vi "PH_PPMA_PowerUnit.ProcCases.vi"(0 "i ref in":refnum<vi>, 1 "selector":string, 2 "Data":T1, 3 "call cluster":T2={"Object"="", "Selector"="", "CallType"=enum."synchronous", "Async Object"="", "Async Selector"="", "Data Descriptor"="", "Data"=[], "Error #"=0, "Expire"=0}, 5 "error in (no error)":errorcluster) -> (14 "i ref out":refnum<vi>, 17 "answer cluster":T2={"Object"="", "Selector"="", "CallType"=enum."synchronous", "Async Object"="", "Async Selector"="", "Data Descriptor"="", "Data"=[], "Error #"=0, "Expire"=0}, 19 "error out":errorcluster)   [LabVIEW 2014, in "PH_PPMA_PowerUnit.lvlib"]
doc: "This method is called by a process from within the default case in the event loop. The methods of a class that are linked to events will be called from THIS method. Add your code here."
uses:
  PH_PPMA_PowerUnit.lvlib
  CSCore/CSSystem/CoreDefs/CoreDefs.call_type.ctl
  CSCore/BaseProcess/BaseProcess.descriptor string definition.ctl
  CSCore/CSSystem/CoreDefs/CoreDefs.rawDataType.ctl
  PH_PowerUnit_BaseClass/PH_PowerUnit_BaseClass.SM States.ctl
  CSCore/CSSystem/CoreLib/CoreLib.string 2 byte array.vi
  CSCore/CSSystem/CoreLib/CoreLib.byte array 2 double.vi
  CSCore/CSSystem/CoreLib/CoreLib.byte array 2 short.vi
  CSCore/CSSystem/CoreLib/CoreLib.lvlib
  CSCore/BaseProcess/BaseProcess.lvlib
  PH_Common/PH_Common.lvlib
  CSCore/CAEObj/CAEObj.lvlib
  lib.lib/DimLVEvent/LVDimInterface/LVDimInterface.lvlib
  PH_StatusHandler/PH_StatusHandler.lvlib
  PH_PSDBWriter/PH_PSDBWriter.lvlib
  CSCore/BaseSM/BaseSM.lvlib
  PH_PowerUnit_BaseClass/PH_PowerUnit_BaseClass.lvlib
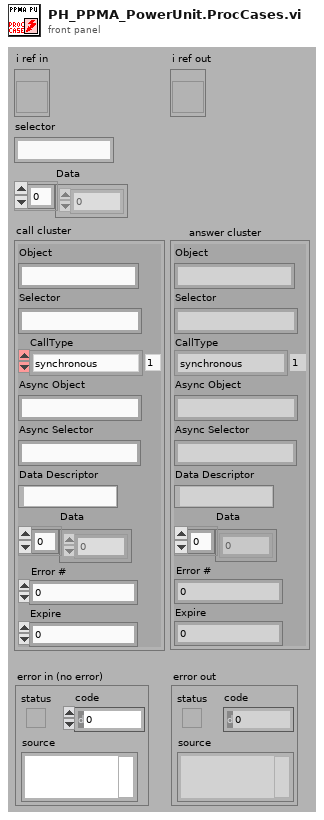
[diagram p1: front panel]
types:
  T1 = typedef "CoreDefs.rawDataType.ctl" = i8[]
  T2 = typedef "CoreDefs.call_type.ctl" = cluster{"Object":string, "Selector":string, "CallType":enum16{"simple", "synchronous", "asynchronous"}, "Async Object":string, "Async Selector":string, "Data Descriptor":T3, "Data":T1, "Error #":i32, "Expire":u32}
  T3 = typedef "BaseProcess.lvlib/BaseProcess.descriptor string definition.ctl" = string
  T4 = typedef "PH_PowerUnit_BaseClass.lvlib/PH_PowerUnit_BaseClass.SM States.ctl" = enum16{".", "Stand by", "Switch PU on", "Configure", "Set Default Voltage", "Set STANDBY", "Set READY", "Wait for Shot Cmd", "Open Dump Rods", "Open Ross Relais", "Close Ross Relais", "Switch PSU on", "Switch PSU off", "Charge", "Switch GD Channel on", "Close Dump Rods", "Rods-TO", "RR-TO", "PSU-TO", "Trigger-TO"}
  T5 = typedef "PH_PowerUnit_BaseClass.lvlib/PH_PowerUnit_BaseClass.i attribute.ctl" = cluster{"Constructor finished":bool, "PU":cluster{"In use":bool, "Service ID in use":i32, "GUI Ref":refnum<vi>}, "Enabling":cluster{"State":T6, "GUI Ref":refnum<vi>}, "Timing":cluster{"Last Shot":dbl, "Time between Shots [Sec]":dbl, "Waiting Time over?":bool, "Service ID Waiting Time":i32, "GUI Ref":refnum<vi>, "Instance":cluster{"Status":T7, "linked?":bool, "GUI Ref":refnum<vi>}}, "Sequencer":cluster{"SM State":string, "GUI Ref":refnum<vi>, "linked":bool}, "Subscribed Trendmssgs":cluster{"Tagname":string, "Status":T7, "linked?":bool, "Shot Condition":T7, "GUI Ref":refnum<vi>}[], "PP PU":T8, "Default Voltage (V)":dbl, "GUI Refs":T9, "PSDB data":cluster{"Shot Voltage [V]":dbl, "State TO SM":T4, "Write 2 early":bool}, "State TO SM":T4}
  T6 = typedef "PH_SystemInformation.lvlib/PH_SystemInformationEnabling State.ctl" = i32
  T7 = typedef "PH_StatusHandler.lvlib/PH_StatusHandler.Status.ctl" = i16
  T8 = typedef "PH_PP_Common.lvlib/PH_PP_Common.PUs.ctl" = enum16{"no Info", "PA-19mm-1", "PA-19mm-2", "PA-45mm-PILC", "PA-45mm-MAIN", "MA-PU-1", "MA-PU-2", "MA-PU-3", "MA-PU-4", "MA-PU-5", "MA-PU-6", "MA-FR", "MA-PILC", "PA-45mm-DP"}
  T9 = typedef "PH_PowerUnit_BaseClass.lvlib/PH_PowerUnit_BaseClass.GUI Refs.ctl" = cluster{"Delete Inst":refnum<vi>, "State TO SM":refnum<vi>, "State SM":refnum<vi>, "Fire":refnum<vi>}
  T10 = typedef "PH_PPMA_PowerUnit.lvlib/PH_PPMA_PowerUnit.i attribute.ctl" = cluster{"GUI Refs":cluster{"Rods":refnum<vi>, "Ignitron":refnum<vi>, "Rossrelais":refnum<vi>, "Set Voltage":refnum<vi>, "PSU":refnum<vi>, "EOC":refnum<vi>, "Trigger":refnum<vi>}, "Rods":T11, "PSU":T12, "Ross Relais":T13, "Ignitron":T14, "Trigger":cluster{"State Device":T7, "linked?":bool}, "Timing Settings":cluster{"Prdc Fast?":bool, "Default Value Periodic Interval":i32, "Mercury on since":dbl, "Warm up Time Mercury [s]":dbl}, "Set Voltage [V]":dbl}
  T11 = typedef "PH_PPMA_PowerUnit.lvlib/PH_PPMA_PowerUnit.Rods Attributes.ctl" = cluster{"Instancename":string, "Device Status":T7, "linked?":bool}
  T12 = typedef "PH_PP_Common.lvlib/PH_PP_Common.PSU Attributes.ctl" = cluster{"lower limit [V]":dbl, "upper limit [V]":dbl, "Voltage set":bool, "State Device":T7, "linked?":bool}
  T13 = typedef "PH_PP_Common.lvlib/PH_PP_Common.Ross Relais Attributes.ctl" = cluster{"State Device":T7, "linked?":bool}
  T14 = typedef "PH_PP_Common.lvlib/PH_PP_Common.Ignitron Attributes.ctl" = cluster{"State Device":T7, "linked?":bool}
  T15 = typedef "PH_PSDBWriter.lvlib/PH_PSDBWriter.PHELIX-Subsystems.ctl" = i32
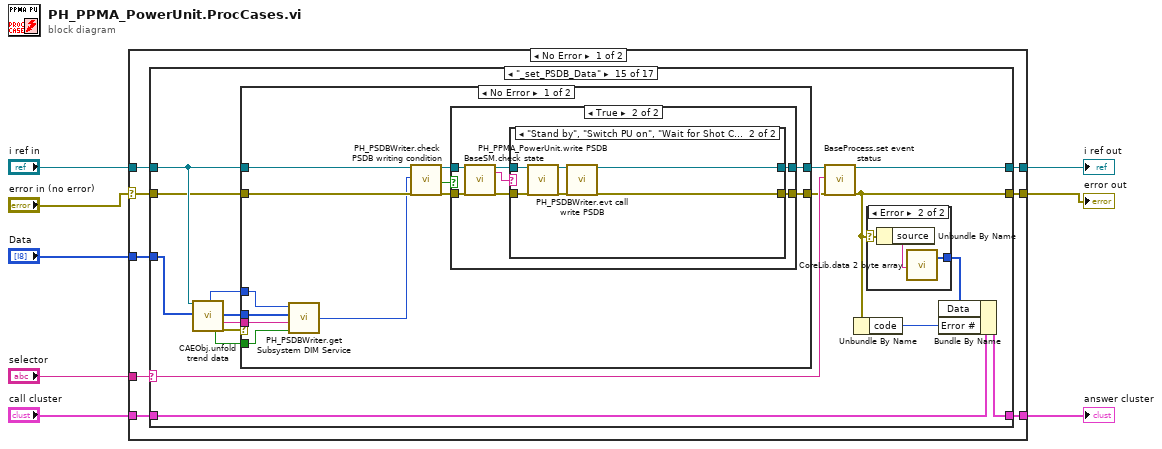
[diagram p0: block diagram]
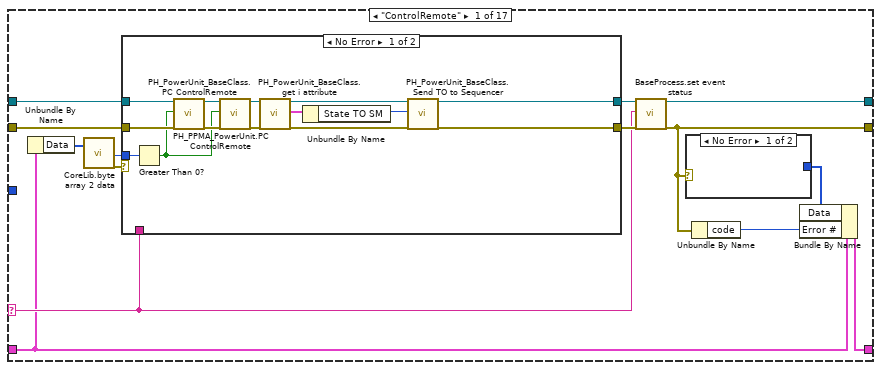
[diagram p2: hidden frame]
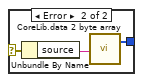
[diagram p3: hidden frame]
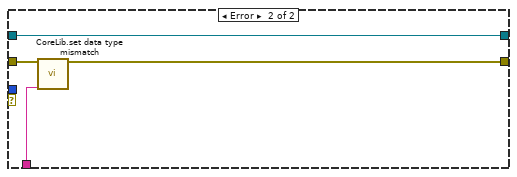
[diagram p4: hidden frame]
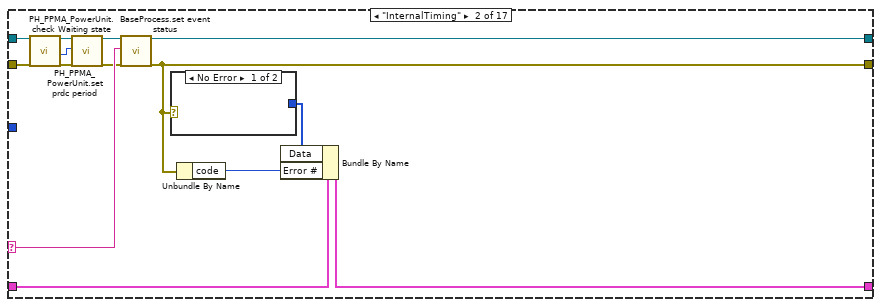
[diagram p5: hidden frame]
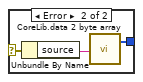
[diagram p6: hidden frame]
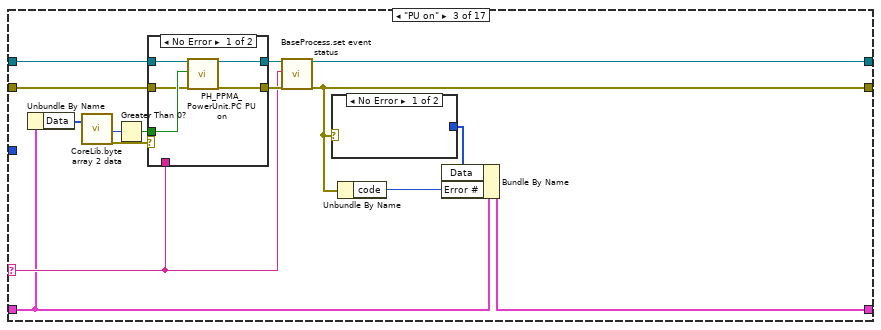
[diagram p7: hidden frame]
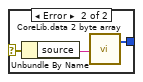
[diagram p8: hidden frame]
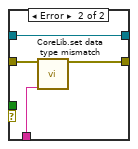
[diagram p9: hidden frame]
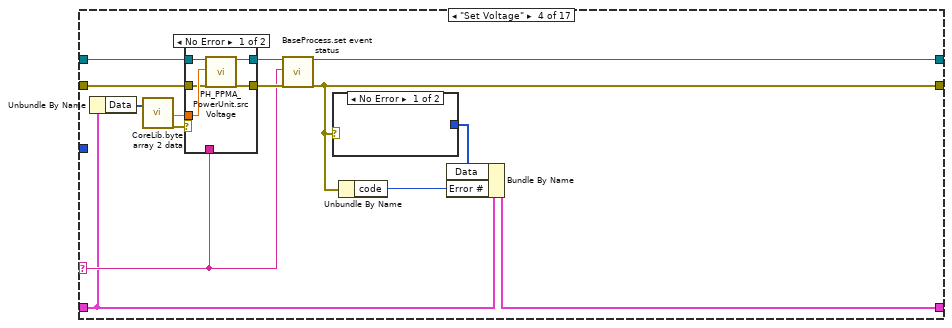
[diagram p10: hidden frame]
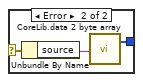
[diagram p11: hidden frame]
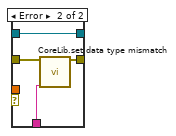
[diagram p12: hidden frame]
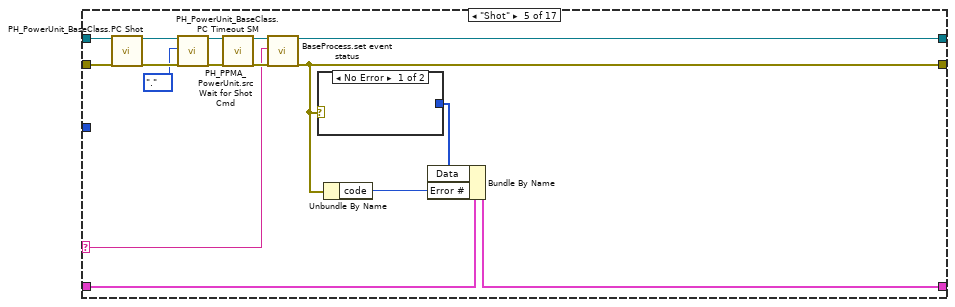
[diagram p13: hidden frame]
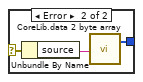
[diagram p14: hidden frame]
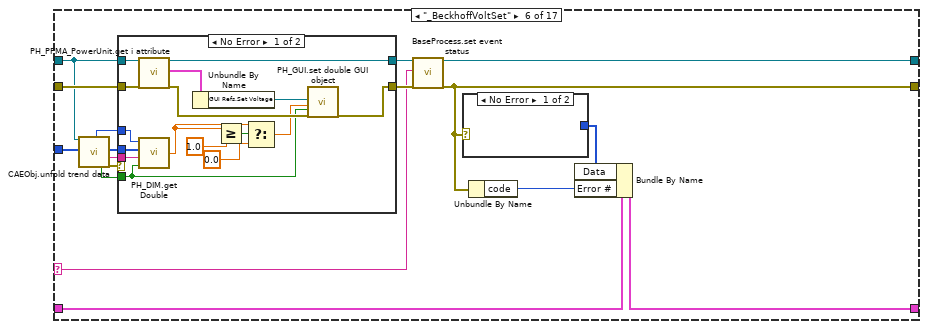
[diagram p15: hidden frame]
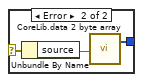
[diagram p16: hidden frame]
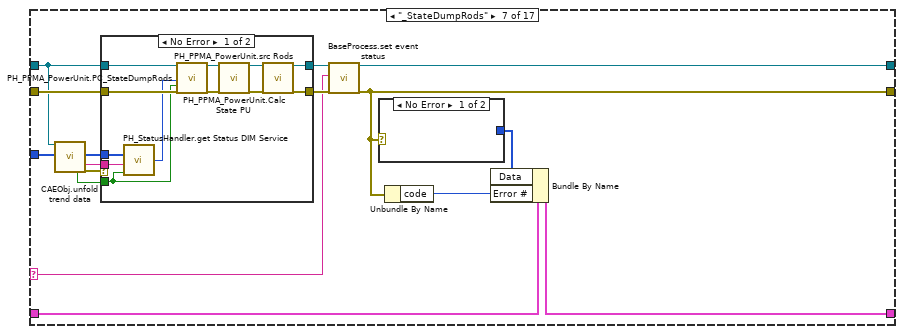
[diagram p18: hidden frame]
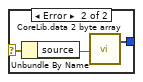
[diagram p19: hidden frame]
diagram:
  n1 = case shown="No Error" "error in (no error)" {
    selector: "error in (no error)" -> [w9 w608]
    tunnel: "selector" -> [w16 _]
    tunnel: [w15 w607] -> w7
    tunnel: "call cluster" -> [w14 w607]
    tunnel: "i ref in" -> [w13 w609]
    tunnel: [w12 w609] -> w4
    tunnel: [w11 w608] -> w3
    tunnel: "Data" -> [w10 _]
    frame No Error {
      n2 = case shown="\"_set_PSDB_Data\"" w16 {
        selector: w16 -> [w19 w61 w71 w98 w127 w143 w181 w217 w246 w299 w341 w376 w409 w444 w510 w576 w603]
        tunnel: w13 -> [w30 w56 w83 w109 w137 w155 w192 w212 w257 w310 w339 w372 w405 w437 w501 w567 w602]
        tunnel: [w21 w63 w74 w100 w123 w145 w183 w213 w248 w301 w345 w378 w411 w446 w512 w578 w599] -> w12
        tunnel: w14 -> [w18 w60 w70 w97 w126 w142 w180 w216 w245 w298 w343 w375 w408 w443 w509 w575 w604]
        tunnel: [w17 w59 w69 w96 w125 w141 w179 w215 w244 w297 w342 w374 w407 w442 w508 w574 w605] -> w15
        tunnel: w9 -> [w29 w57 w82 w108 w136 w157 w194 w227 w259 w312 w350 w383 w416 w438 w500 w566 w606]
        tunnel: [w20 w62 w72 w99 w124 w144 w182 w214 w247 w300 w344 w377 w410 w445 w511 w577 w597] -> w11
        tunnel: w10 -> [_ _ _ _ _ w156 w193 w226 w258 w311 w340 w373 w406 w434 w502 w568 w601]
        frame "ControlRemote" {
          n3 = Unbundle By Name(w18) -> ("Data"=w28:T1)
          n4 = call-poly "CoreLib.byte array 2 data.vi"("byteArray"=w28) -> ("i16"=w27:i16, "error out"=w26:errorcluster)  [unwired: 16 in, 1 out]
          n5 = case shown="No Error" w26 {
            tunnel: [w36 w51] -> w23
            tunnel: w30 -> [w47 w51]
            tunnel: w29 -> [w46 w50]
            tunnel: [w35 w49] -> w22
            tunnel: w19 -> [_ w48]
            tunnel: w27 -> [w45 _]
            frame No Error {
              n6 = Greater Than 0?(x=w45) -> (x > 0?=w38:bool)
              n7 = call "PH_PPMA_PowerUnit.PC ControlRemote.vi"("i ref in"=w47, "Remote controlled?"=w38, "error in (no error)"=w46) -> ("i ref out"=w42:refnum<vi>, "error out"=w40:errorcluster)  [unwired: 15 in]
              n8 = call "PH_PowerUnit_BaseClass.PC ControlRemote.vi"("i ref in"=w42, "Remote controlled?"=w38, "error in (no error)"=w40) -> ("i ref out"=w41:refnum<vi>, "error out"=w39:errorcluster)  [unwired: 15 in]
              n9 = call "PH_PowerUnit_BaseClass.get i attribute.vi"("i ref in"=w41, "error in (no error)"=w39) -> ("i ref out"=w37:refnum<vi>, "i attribute"=w44:T5, "error out"=w43:errorcluster)  [unwired: 15 in]
              n10 = Unbundle By Name(w44) -> ("State TO SM"=w34:T4)
              n11 = call "PH_PowerUnit_BaseClass.Send TO to Sequencer.vi"("VI in"=w37, "State TO SM"=w34, "error in (no error)"=w43) -> ("VI out"=w36:refnum<vi>, "error out"=w35:errorcluster)  [unwired: 15 in]
            }
            frame Error {
              n12 = call "CoreLib.set data type mismatch.vi"("error in (no error)"=w50, "error source"=w48) -> ("error out"=w49:errorcluster)  [unwired: 17 in]
            }
          }
          n13 = call "BaseProcess.set event status.vi"("i ref in"=w23, "EventStatus"=w19, "error in (no error)"=w22) -> ("i ref out"=w21:refnum<vi>, "error out"=w20:errorcluster)  [unwired: 14 in, 1 out]
          n14 = case shown="No Error" w20 {
            selector: w20 -> [_ w33]
            tunnel: [_ w31] -> w24
            frame No Error {
            }
            frame Error {
              n15 = Unbundle By Name(w33) -> ("source"=w32:string)
              n16 = call-poly "CoreLib.data 2 byte array.vi"("string"=w32) -> ("byteArray out"=w31:T1)  [unwired: 18 in]
            }
          }
          n17 = Unbundle By Name(w20) -> ("code"=w25:i32)
          n18 = Bundle By Name(cluster=w18, "Data"=w24, "Error #"=w25) -> (w17:T2)
        }
        frame "InternalTiming" {
          n19 = call "PH_PPMA_PowerUnit.check Waiting state.vi"("i ref in"=w56, "error in (no error)"=w57) -> ("i ref out"=w53:refnum<vi>, "Waiting Time (s)"=w58:i32, "error out"=w52:errorcluster)  [unwired: 15 in]
          n20 = call "PH_PPMA_PowerUnit.set  prdc period.vi"("i ref in"=w53, "Waiting Time (s)"=w58, "error in (no error)"=w52) -> ("i ref out"=w55:refnum<vi>, "error out"=w54:errorcluster)  [unwired: 15 in]
          n21 = call "BaseProcess.set event status.vi"("i ref in"=w55, "EventStatus"=w61, "error in (no error)"=w54) -> ("i ref out"=w63:refnum<vi>, "error out"=w62:errorcluster)  [unwired: 14 in, 1 out]
          n22 = case shown="No Error" w62 {
            selector: w62 -> [_ w68]
            tunnel: [_ w66] -> w64
            frame No Error {
            }
            frame Error {
              n23 = Unbundle By Name(w68) -> ("source"=w67:string)
              n24 = call-poly "CoreLib.data 2 byte array.vi"("string"=w67) -> ("byteArray out"=w66:T1)  [unwired: 18 in]
            }
          }
          n25 = Unbundle By Name(w62) -> ("code"=w65:i32)
          n26 = Bundle By Name(cluster=w60, "Data"=w64, "Error #"=w65) -> (w59:T2)
        }
        frame "PU on" {
          n27 = Unbundle By Name(w70) -> ("Data"=w80:T1)
          n28 = call-poly "CoreLib.byte array 2 data.vi"("byteArray"=w80) -> ("i16"=w81:i16, "error out"=w78:errorcluster)  [unwired: 16 in, 1 out]
          n29 = Greater Than 0?(x=w81) -> (x > 0?=w79:bool)
          n30 = case shown="No Error" w78 {
            tunnel: [w91 w95] -> w75
            tunnel: w83 -> [w88 w95]
            tunnel: w82 -> [w87 w94]
            tunnel: [w90 w93] -> w73
            tunnel: w71 -> [_ w92]
            tunnel: w79 -> [w89 _]
            frame No Error {
              n31 = call "PH_PPMA_PowerUnit.PC PU on.vi"("i ref in"=w88, "PU on"=w89, "error in (no error)"=w87) -> ("i ref out"=w91:refnum<vi>, "error out"=w90:errorcluster)  [unwired: 15 in]
            }
            frame Error {
              n32 = call "CoreLib.set data type mismatch.vi"("error in (no error)"=w94, "error source"=w92) -> ("error out"=w93:errorcluster)  [unwired: 17 in]
            }
          }
          n33 = call "BaseProcess.set event status.vi"("i ref in"=w75, "EventStatus"=w71, "error in (no error)"=w73) -> ("i ref out"=w74:refnum<vi>, "error out"=w72:errorcluster)  [unwired: 14 in, 1 out]
          n34 = case shown="No Error" w72 {
            selector: w72 -> [_ w86]
            tunnel: [_ w84] -> w76
            frame No Error {
            }
            frame Error {
              n35 = Unbundle By Name(w86) -> ("source"=w85:string)
              n36 = call-poly "CoreLib.data 2 byte array.vi"("string"=w85) -> ("byteArray out"=w84:T1)  [unwired: 18 in]
            }
          }
          n37 = Unbundle By Name(w72) -> ("code"=w77:i32)
          n38 = Bundle By Name(cluster=w70, "Data"=w76, "Error #"=w77) -> (w69:T2)
        }
        frame "Set Voltage" {
          n39 = Unbundle By Name(w97) -> ("Data"=w107:T1)
          n40 = call-poly "CoreLib.byte array 2 data.vi"("byteArray"=w107) -> ("d64"=w105:dbl, "error out"=w106:errorcluster)  [unwired: 16 in, 1 out]
          n41 = case shown="No Error" w106 {
            tunnel: [w116 w121] -> w101
            tunnel: w109 -> [w114 w121]
            tunnel: w108 -> [w113 w120]
            tunnel: [w117 w119] -> w102
            tunnel: w98 -> [_ w118]
            tunnel: w105 -> [w115 _]
            frame No Error {
              n42 = call "PH_PPMA_PowerUnit.src Voltage.vi"("i ref in"=w114, "Voltage [V]"=w115, "error in (no error)"=w113) -> ("i ref out"=w116:refnum<vi>, "error out"=w117:errorcluster)  [unwired: 15 in]
            }
            frame Error {
              n43 = call "CoreLib.set data type mismatch.vi"("error in (no error)"=w120, "error source"=w118) -> ("error out"=w119:errorcluster)  [unwired: 17 in]
            }
          }
          n44 = call "BaseProcess.set event status.vi"("i ref in"=w101, "EventStatus"=w98, "error in (no error)"=w102) -> ("i ref out"=w100:refnum<vi>, "error out"=w99:errorcluster)  [unwired: 14 in, 1 out]
          n45 = case shown="No Error" w99 {
            selector: w99 -> [_ w112]
            tunnel: [_ w110] -> w103
            frame No Error {
            }
            frame Error {
              n46 = Unbundle By Name(w112) -> ("source"=w111:string)
              n47 = call-poly "CoreLib.data 2 byte array.vi"("string"=w111) -> ("byteArray out"=w110:T1)  [unwired: 18 in]
            }
          }
          n48 = Unbundle By Name(w99) -> ("code"=w104:i32)
          n49 = Bundle By Name(cluster=w97, "Data"=w103, "Error #"=w104) -> (w96:T2)
        }
        frame "Shot" {
          n50 = call "PH_PowerUnit_BaseClass.PC Shot.vi"("i ref in"=w137, "error in (no error)"=w136) -> ("i ref out"=w135:refnum<vi>, "error out"=w134:errorcluster)  [unwired: 16 in]
          n51 = call "PH_PowerUnit_BaseClass.PC Timeout SM.vi"("VI in"=w135, "Timeout SM"=PH_PowerUnit_BaseClass.SM_States.".", "error in (no error)"=w134) -> ("VI out"=w132:refnum<vi>, "error out"=w133:errorcluster)  [unwired: 15 in]
          n52 = call "PH_PPMA_PowerUnit.src Wait for Shot Cmd.vi"("i ref in"=w132, "error in (no error)"=w133) -> ("i ref out"=w129:refnum<vi>, "error out"=w128:errorcluster)  [unwired: 16 in]
          n53 = call "BaseProcess.set event status.vi"("i ref in"=w129, "EventStatus"=w127, "error in (no error)"=w128) -> ("i ref out"=w123:refnum<vi>, "error out"=w124:errorcluster)  [unwired: 14 in, 1 out]
          n54 = case shown="No Error" w124 {
            selector: w124 -> [_ w140]
            tunnel: [_ w138] -> w130
            frame No Error {
            }
            frame Error {
              n55 = Unbundle By Name(w140) -> ("source"=w139:string)
              n56 = call-poly "CoreLib.data 2 byte array.vi"("string"=w139) -> ("byteArray out"=w138:T1)  [unwired: 18 in]
            }
          }
          n57 = Unbundle By Name(w124) -> ("code"=w131:i32)
          n58 = Bundle By Name(cluster=w126, "Data"=w130, "Error #"=w131) -> (w125:T2)
        }
        frame "_BeckhoffVoltSet" {
          n59 = call "CAEObj.unfold trend data.vi"("i ref in"=w155, "raw trend data"=w156) -> ("quality"=w151:i32, "no link"=w152:bool, "data"=w153:i8[], "typeDescriptor"=w150:string, "error out"=w154:errorcluster)  [unwired: 9 in, 4 out]
          n60 = case shown="No Error" w154 {
            tunnel: w155 -> [w176 w178]
            tunnel: [w173 w178] -> w146
            tunnel: w157 -> [w175 w177]
            tunnel: [w164 w177] -> w147
            tunnel: w153 -> [w168 _]
            tunnel: w152 -> [w161 _]
            tunnel: w151 -> [w167 _]
            tunnel: w150 -> [w166 _]
            frame No Error {
              n61 = call "PH_PPMA_PowerUnit.get i attribute.vi"("i ref in"=w176, "error in (no error)"=w175) -> ("i ref out"=w173:refnum<vi>, "i attribute"=w174:T10, "error out"=w165:errorcluster)  [unwired: 15 in]
              n62 = call "PH_DIM.get Double.vi"("no link"=w161, "typeDescriptor"=w166, "data"=w168, "quality"=w167) -> ("Value"=w171:dbl)
              n63 = Unbundle By Name(w174) -> ("GUI Refs.Set Voltage"=w163:refnum<vi>)
              n64 = Greater Or Equal?(x=w171, y=1.0) -> (x >= y?=w172:bool)
              n65 = Select(t=w171, s=w172, f=0.0) -> (s? t:f=w162:dbl)
              n66 = call "PH_GUI.set double GUI object.vi"("GUI object Ref"=w163, "value"=w162, "blinking (false)"=w161, "error in (no error)"=w165) -> ("error out"=w164:errorcluster)  [unwired: 15 in]
            }
            frame Error {
            }
          }
          n67 = call "BaseProcess.set event status.vi"("i ref in"=w146, "EventStatus"=w143, "error in (no error)"=w147) -> ("i ref out"=w145:refnum<vi>, "error out"=w144:errorcluster)  [unwired: 14 in, 1 out]
          n68 = case shown="No Error" w144 {
            selector: w144 -> [_ w160]
            tunnel: [_ w158] -> w148
            frame No Error {
            }
            frame Error {
              n69 = Unbundle By Name(w160) -> ("source"=w159:string)
              n70 = call-poly "CoreLib.data 2 byte array.vi"("string"=w159) -> ("byteArray out"=w158:T1)  [unwired: 18 in]
            }
          }
          n71 = Unbundle By Name(w144) -> ("code"=w149:i32)
          n72 = Bundle By Name(cluster=w142, "Data"=w148, "Error #"=w149) -> (w141:T2)
        }
        frame "_StateDumpRods" {
          n73 = call "CAEObj.unfold trend data.vi"("i ref in"=w192, "raw trend data"=w193) -> ("no link"=w188:bool, "data"=w189:i8[], "typeDescriptor"=w190:string, "error out"=w191:errorcluster)  [unwired: 9 in, 5 out]
          n74 = case shown="No Error" w191 {
            tunnel: w192 -> [w209 w211]
            tunnel: [w202 w211] -> w184
            tunnel: w194 -> [w208 w210]
            tunnel: [w203 w210] -> w185
            tunnel: w190 -> [w207 _]
            tunnel: w189 -> [w206 _]
            tunnel: w188 -> [w204 _]
            frame No Error {
              n75 = call "PH_StatusHandler.get Status DIM Service.vi"("no link"=w204, "typeDescriptor"=w207, "data"=w206) -> ("Status"=w205:T7)  [unwired: 1 in]
              n76 = call "PH_PPMA_PowerUnit.PC_StateDumpRods.vi"("i ref in"=w209, "Rods Status"=w205, "not linked?"=w204, "error in (no error)"=w208) -> ("i ref out"=w201:refnum<vi>, "error out"=w199:errorcluster)  [unwired: 14 in]
              n77 = call "PH_PPMA_PowerUnit.Calc State PU.vi"("i ref in"=w201, "error in (no error)"=w199) -> ("i ref out"=w200:refnum<vi>, "error out"=w198:errorcluster)  [unwired: 16 in]
              n78 = call "PH_PPMA_PowerUnit.src Rods.vi"("i ref in"=w200, "error in (no error)"=w198) -> ("i ref out"=w202:refnum<vi>, "error out"=w203:errorcluster)  [unwired: 16 in]
            }
            frame Error {
            }
          }
          n79 = call "BaseProcess.set event status.vi"("i ref in"=w184, "EventStatus"=w181, "error in (no error)"=w185) -> ("i ref out"=w183:refnum<vi>, "error out"=w182:errorcluster)  [unwired: 14 in, 1 out]
          n80 = case shown="No Error" w182 {
            selector: w182 -> [_ w197]
            tunnel: [_ w195] -> w186
            frame No Error {
            }
            frame Error {
              n81 = Unbundle By Name(w197) -> ("source"=w196:string)
              n82 = call-poly "CoreLib.data 2 byte array.vi"("string"=w196) -> ("byteArray out"=w195:T1)  [unwired: 18 in]
            }
          }
          n83 = Unbundle By Name(w182) -> ("code"=w187:i32)
          n84 = Bundle By Name(cluster=w180, "Data"=w186, "Error #"=w187) -> (w179:T2)
        }
        frame "_StateIgni" {
          n85 = call "CAEObj.unfold trend data.vi"("i ref in"=w212, "raw trend data"=w226) -> ("no link"=w222:bool, "data"=w223:i8[], "typeDescriptor"=w224:string, "error out"=w225:errorcluster)  [unwired: 9 in, 5 out]
          n86 = case shown="No Error" w225 {
            tunnel: w212 -> [w240 w242]
            tunnel: [w237 w242] -> w219
            tunnel: w227 -> [w239 w241]
            tunnel: [w238 w241] -> w218
            tunnel: w224 -> [w234 _]
            tunnel: w223 -> [w233 _]
            tunnel: w222 -> [w231 _]
            frame No Error {
              n87 = call "PH_StatusHandler.get Status DIM Service.vi"("no link"=w231, "typeDescriptor"=w234, "data"=w233) -> ("Status"=w232:T7)  [unwired: 1 in]
              n88 = call "PH_PPMA_PowerUnit.PC_StateIgni.vi"("i ref in"=w240, "Ignitron Status"=w232, "not linked?"=w231, "error in (no error)"=w239) -> ("i ref out"=w235:refnum<vi>, "error out"=w236:errorcluster)  [unwired: 14 in]
              n89 = call "PH_PPMA_PowerUnit.Calc State PU.vi"("i ref in"=w235, "error in (no error)"=w236) -> ("i ref out"=w237:refnum<vi>, "error out"=w238:errorcluster)  [unwired: 16 in]
            }
            frame Error {
            }
          }
          n90 = call "BaseProcess.set event status.vi"("i ref in"=w219, "EventStatus"=w217, "error in (no error)"=w218) -> ("i ref out"=w213:refnum<vi>, "error out"=w214:errorcluster)  [unwired: 14 in, 1 out]
          n91 = case shown="No Error" w214 {
            selector: w214 -> [_ w230]
            tunnel: [_ w228] -> w220
            frame No Error {
            }
            frame Error {
              n92 = Unbundle By Name(w230) -> ("source"=w229:string)
              n93 = call-poly "CoreLib.data 2 byte array.vi"("string"=w229) -> ("byteArray out"=w228:T1)  [unwired: 18 in]
            }
          }
          n94 = Unbundle By Name(w214) -> ("code"=w221:i32)
          n95 = Bundle By Name(cluster=w216, "Data"=w220, "Error #"=w221) -> (w215:T2)
        }
        frame "_MercuryOnSince" {
          n96 = call "CAEObj.unfold trend data.vi"("i ref in"=w257, "raw trend data"=w258) -> ("quality"=w243:i32, "no link"=w253:bool, "data"=w255:i8[], "typeDescriptor"=w254:string, "error out"=w256:errorcluster)  [unwired: 9 in, 4 out]
          n97 = case shown="No Error" w256 {
            tunnel: w257 -> [w275 w295]
            tunnel: [w270 w295] -> w249
            tunnel: w259 -> [w274 w294]
            tunnel: [w268 w294] -> w250
            tunnel: w255 -> [w273 _]
            tunnel: w254 -> [w272 _]
            tunnel: w253 -> [w263 _]
            tunnel: w243 -> [w267 _]
            frame No Error {
              n98 = call "PH_PPMA_PowerUnit.get data to modify.vi"("i ref in"=w275, "error in (no error)"=w274) -> ("i ref out"=w271:refnum<vi>, "i attribute"=w264:T10, "timed out"=w265:bool, "error out"=w269:errorcluster)  [unwired: 14 in]
              n99 = call "PH_DIM.get String.vi"("no link"=w263, "typeDescriptor"=w272, "data"=w273, "quality"=w267) -> ("Output String"=w266:string)
              n100 = case shown="False" w265 {
                tunnel: w271 -> [w284 w293]
                tunnel: [w283 w293] -> w270
                tunnel: w269 -> [w282 w292]
                tunnel: [w281 w292] -> w268
                tunnel: w266 -> [w280 _]
                tunnel: w264 -> [w279 _]
                tunnel: w263 -> [w277 _]
                frame False {
                  n101 = case shown="False" w277 {
                    tunnel: w280 -> [w287 _]
                    tunnel: [w286 9999.0] -> w276
                    frame False {
                      n102 = Match Pattern(string=w287, regular expression=" ") -> (before substring=w289:string, after substring=w288:string)  [unwired: 1 in, 2 out]
                      n103 = call "PH_Strings.convert Time 1.vi"("Date"=w289, "Time"=w288) -> ("Time"=w285:timestamp)
                      n104 = To Double Precision Float(number=w285) -> (double precision float=w286:dbl)
                    }
                    frame True {
                    }
                  }
                  n105 = Bundle By Name(cluster=w279, "Timing Settings.Mercury on since"=w276) -> (w278:T10)
                  n106 = call "PH_PPMA_PowerUnit.set modified data.vi"("i ref in"=w284, "i attribute"=w278, "error in (no error)"=w282) -> ("i ref out"=w283:refnum<vi>, "error out"=w281:errorcluster)  [unwired: 15 in]
                }
                frame True {
                }
              }
            }
            frame Error {
            }
          }
          n107 = call "BaseProcess.set event status.vi"("i ref in"=w249, "EventStatus"=w246, "error in (no error)"=w250) -> ("i ref out"=w248:refnum<vi>, "error out"=w247:errorcluster)  [unwired: 14 in, 1 out]
          n108 = case shown="No Error" w247 {
            selector: w247 -> [_ w262]
            tunnel: [_ w260] -> w251
            frame No Error {
            }
            frame Error {
              n109 = Unbundle By Name(w262) -> ("source"=w261:string)
              n110 = call-poly "CoreLib.data 2 byte array.vi"("string"=w261) -> ("byteArray out"=w260:T1)  [unwired: 18 in]
            }
          }
          n111 = Unbundle By Name(w247) -> ("code"=w252:i32)
          n112 = Bundle By Name(cluster=w245, "Data"=w251, "Error #"=w252) -> (w244:T2)
        }
        frame "_LastShot" {
          n113 = call "CAEObj.unfold trend data.vi"("i ref in"=w310, "raw trend data"=w311) -> ("quality"=w296:i32, "no link"=w306:bool, "data"=w308:i8[], "typeDescriptor"=w307:string, "error out"=w309:errorcluster)  [unwired: 9 in, 4 out]
          n114 = case shown="No Error" w309 {
            tunnel: w310 -> [w317 w334]
            tunnel: [w323 w334] -> w302
            tunnel: w312 -> [w316 w333]
            tunnel: [w322 w333] -> w303
            tunnel: w308 -> [w325 _]
            tunnel: w307 -> [w324 _]
            tunnel: w306 -> [w319 _]
            tunnel: w296 -> [w321 _]
            frame No Error {
              n115 = call "PH_DIM.get String.vi"("no link"=w319, "typeDescriptor"=w324, "data"=w325, "quality"=w321) -> ("Output String"=w320:string)
              n116 = case shown="False" w319 {
                tunnel: w320 -> [w328 _]
                tunnel: [w326 9999.0] -> w318
                frame False {
                  n117 = Match Pattern(string=w328, regular expression=" ") -> (before substring=w330:string, after substring=w329:string)  [unwired: 1 in, 2 out]
                  n118 = call "PH_Strings.convert Time 1.vi"("Date"=w330, "Time"=w329) -> ("Time"=w327:timestamp)
                  n119 = To Double Precision Float(number=w327) -> (double precision float=w326:dbl)
                }
                frame True {
                }
              }
              n120 = call "PH_PowerUnit_BaseClass.set Last Shot.vi"("VI in"=w317, "Last Shot"=w318, "error in (no error)"=w316) -> ("VI out"=w323:refnum<vi>, "error out"=w322:errorcluster)  [unwired: 15 in]
            }
            frame Error {
            }
          }
          n121 = call "BaseProcess.set event status.vi"("i ref in"=w302, "EventStatus"=w299, "error in (no error)"=w303) -> ("i ref out"=w301:refnum<vi>, "error out"=w300:errorcluster)  [unwired: 14 in, 1 out]
          n122 = case shown="No Error" w300 {
            selector: w300 -> [_ w315]
            tunnel: [_ w313] -> w304
            frame No Error {
            }
            frame Error {
              n123 = Unbundle By Name(w315) -> ("source"=w314:string)
              n124 = call-poly "CoreLib.data 2 byte array.vi"("string"=w314) -> ("byteArray out"=w313:T1)  [unwired: 18 in]
            }
          }
          n125 = Unbundle By Name(w300) -> ("code"=w305:i32)
          n126 = Bundle By Name(cluster=w298, "Data"=w304, "Error #"=w305) -> (w297:T2)
        }
        frame "_StatePSU" {
          n127 = call "CAEObj.unfold trend data.vi"("i ref in"=w339, "raw trend data"=w340) -> ("no link"=w335:bool, "data"=w336:i8[], "typeDescriptor"=w337:string, "error out"=w338:errorcluster)  [unwired: 9 in, 5 out]
          n128 = case shown="No Error" w338 {
            tunnel: w339 -> [w365 w367]
            tunnel: [w363 w367] -> w347
            tunnel: w350 -> [w364 w366]
            tunnel: [w362 w366] -> w346
            tunnel: w337 -> [w361 _]
            tunnel: w336 -> [w360 _]
            tunnel: w335 -> [w358 _]
            frame No Error {
              n129 = call "PH_StatusHandler.get Status DIM Service.vi"("no link"=w358, "typeDescriptor"=w361, "data"=w360) -> ("Status"=w359:T7)  [unwired: 1 in]
              n130 = call "PH_PPMA_PowerUnit.PC_StatePSU.vi"("i ref in"=w365, "PSU Status"=w359, "not linked?"=w358, "error in (no error)"=w364) -> ("i ref out"=w355:refnum<vi>, "error out"=w357:errorcluster)  [unwired: 14 in]
              n131 = call "PH_PPMA_PowerUnit.Calc State PU.vi"("i ref in"=w355, "error in (no error)"=w357) -> ("i ref out"=w354:refnum<vi>, "error out"=w356:errorcluster)  [unwired: 16 in]
              n132 = call "PH_PPMA_PowerUnit.src PSU.vi"("i ref in"=w354, "error in (no error)"=w356) -> ("i ref out"=w363:refnum<vi>, "error out"=w362:errorcluster)  [unwired: 16 in]
            }
            frame Error {
            }
          }
          n133 = call "BaseProcess.set event status.vi"("i ref in"=w347, "EventStatus"=w341, "error in (no error)"=w346) -> ("i ref out"=w345:refnum<vi>, "error out"=w344:errorcluster)  [unwired: 14 in, 1 out]
          n134 = case shown="Error" w344 {
            selector: w344 -> [_ w353]
            tunnel: [_ w351] -> w348
            frame No Error {
            }
            frame Error {
              n135 = Unbundle By Name(w353) -> ("source"=w352:string)
              n136 = call-poly "CoreLib.data 2 byte array.vi"("string"=w352) -> ("byteArray out"=w351:T1)  [unwired: 18 in]
            }
          }
          n137 = Unbundle By Name(w344) -> ("code"=w349:i32)
          n138 = Bundle By Name(cluster=w343, "Data"=w348, "Error #"=w349) -> (w342:T2)
        }
        frame "_StateRoss" {
          n139 = call "CAEObj.unfold trend data.vi"("i ref in"=w372, "raw trend data"=w373) -> ("no link"=w368:bool, "data"=w370:i8[], "typeDescriptor"=w369:string, "error out"=w371:errorcluster)  [unwired: 9 in, 5 out]
          n140 = case shown="No Error" w371 {
            tunnel: w372 -> [w398 w400]
            tunnel: [w396 w400] -> w379
            tunnel: w383 -> [w397 w399]
            tunnel: [w395 w399] -> w380
            tunnel: w370 -> [w394 _]
            tunnel: w369 -> [w393 _]
            tunnel: w368 -> [w391 _]
            frame No Error {
              n141 = call "PH_StatusHandler.get Status DIM Service.vi"("no link"=w391, "typeDescriptor"=w393, "data"=w394) -> ("Status"=w392:T7)  [unwired: 1 in]
              n142 = call "PH_PPMA_PowerUnit.PC_StateRoss.vi"("i ref in"=w398, "Ross Status"=w392, "not linked?"=w391, "error in (no error)"=w397) -> ("i ref out"=w390:refnum<vi>, "error out"=w388:errorcluster)  [unwired: 14 in]
              n143 = call "PH_PPMA_PowerUnit.Calc State PU.vi"("i ref in"=w390, "error in (no error)"=w388) -> ("i ref out"=w389:refnum<vi>, "error out"=w387:errorcluster)  [unwired: 16 in]
              n144 = call "PH_PPMA_PowerUnit.src Ross.vi"("i ref in"=w389, "error in (no error)"=w387) -> ("i ref out"=w396:refnum<vi>, "error out"=w395:errorcluster)  [unwired: 16 in]
            }
            frame Error {
            }
          }
          n145 = call "BaseProcess.set event status.vi"("i ref in"=w379, "EventStatus"=w376, "error in (no error)"=w380) -> ("i ref out"=w378:refnum<vi>, "error out"=w377:errorcluster)  [unwired: 14 in, 1 out]
          n146 = case shown="Error" w377 {
            selector: w377 -> [_ w386]
            tunnel: [_ w384] -> w381
            frame No Error {
            }
            frame Error {
              n147 = Unbundle By Name(w386) -> ("source"=w385:string)
              n148 = call-poly "CoreLib.data 2 byte array.vi"("string"=w385) -> ("byteArray out"=w384:T1)  [unwired: 18 in]
            }
          }
          n149 = Unbundle By Name(w377) -> ("code"=w382:i32)
          n150 = Bundle By Name(cluster=w375, "Data"=w381, "Error #"=w382) -> (w374:T2)
        }
        frame "_StateTrigger" {
          n151 = call "CAEObj.unfold trend data.vi"("i ref in"=w405, "raw trend data"=w406) -> ("no link"=w401:bool, "data"=w403:i8[], "typeDescriptor"=w402:string, "error out"=w404:errorcluster)  [unwired: 9 in, 5 out]
          n152 = case shown="No Error" w404 {
            tunnel: w405 -> [w431 w433]
            tunnel: [w429 w433] -> w412
            tunnel: w416 -> [w430 w432]
            tunnel: [w428 w432] -> w413
            tunnel: w403 -> [w427 _]
            tunnel: w402 -> [w426 _]
            tunnel: w401 -> [w424 _]
            frame No Error {
              n153 = call "PH_StatusHandler.get Status DIM Service.vi"("no link"=w424, "typeDescriptor"=w426, "data"=w427) -> ("Status"=w425:T7)  [unwired: 1 in]
              n154 = call "PH_PPMA_PowerUnit.PC_StateTrigger.vi"("i ref in"=w431, "State Trigger"=w425, "not linked?"=w424, "error in (no error)"=w430) -> ("i ref out"=w423:refnum<vi>, "error out"=w421:errorcluster)  [unwired: 14 in]
              n155 = call "PH_PPMA_PowerUnit.Calc State PU.vi"("i ref in"=w423, "error in (no error)"=w421) -> ("i ref out"=w422:refnum<vi>, "error out"=w420:errorcluster)  [unwired: 16 in]
              n156 = call "PH_PPMA_PowerUnit.src Switch GD Channel on.vi"("i ref in"=w422, "error in (no error)"=w420) -> ("i ref out"=w429:refnum<vi>, "error out"=w428:errorcluster)  [unwired: 16 in]
            }
            frame Error {
            }
          }
          n157 = call "BaseProcess.set event status.vi"("i ref in"=w412, "EventStatus"=w409, "error in (no error)"=w413) -> ("i ref out"=w411:refnum<vi>, "error out"=w410:errorcluster)  [unwired: 14 in, 1 out]
          n158 = case shown="Error" w410 {
            selector: w410 -> [_ w419]
            tunnel: [_ w417] -> w414
            frame No Error {
            }
            frame Error {
              n159 = Unbundle By Name(w419) -> ("source"=w418:string)
              n160 = call-poly "CoreLib.data 2 byte array.vi"("string"=w418) -> ("byteArray out"=w417:T1)  [unwired: 18 in]
            }
          }
          n161 = Unbundle By Name(w410) -> ("code"=w415:i32)
          n162 = Bundle By Name(cluster=w408, "Data"=w414, "Error #"=w415) -> (w407:T2)
        }
        frame "_getLimits" {
          n163 = call "LVDimInterface.dim_unfold_data.vi"("rawData"=w434) -> ("data"=w441:i8[], "no link"=w439:bool, "error out"=w440:errorcluster)  [unwired: 15 in, 1 out]
          n164 = case shown="No Error" w440 {
            tunnel: w437 -> [w463 w494]
            tunnel: [w461 w494] -> w436
            tunnel: w438 -> [w453 w493]
            tunnel: [w459 w493] -> w435
            tunnel: w441 -> [w451 _]
            tunnel: w439 -> [w464 _]
            frame No Error {
              n165 = call "PH_PowerUnit_BaseClass.get i attribute.vi"("i ref in"=w463, "error in (no error)"=w453) -> ("i ref out"=w454:refnum<vi>, "i attribute"=w450:T5, "error out"=w452:errorcluster)  [unwired: 15 in]
              n166 = Unbundle By Name(w450) -> ("PP PU"=w449:T8)
              n167 = case shown="False" w464 {
                tunnel: [w478 w492] -> w457
                tunnel: [w477 w492] -> w456
                tunnel: w451 -> [w476 _]
                tunnel: w449 -> [w475 _]
                frame False {
                  n168 = case shown="Default" w475 {
                    tunnel: [w483 w488] -> w478
                    tunnel: [w482 w487] -> w477
                    tunnel: w476 -> [w479 w491]
                    frame Default {
                      n169 = Type Cast(type="", x=w479) -> (*(type *) &x=w480:string)
                      n170 = call "CoreLib.stringToStringArray.vi"("String"=w480) -> ("Array"=w486:string[])
                      n171 = Index Array(array=w486) -> (element #1=w485:string, element #2=w484:string)  [unwired: 2 in]
                      n172 = Fract/Exp String To Number(string=w485) -> (number=w483:dbl)  [unwired: 3 in, 1 out]
                      n173 = Fract/Exp String To Number(string=w484) -> (number=w482:dbl)  [unwired: 3 in, 1 out]
                    }
                    frame "MA-PU-1".."MA-PILC" {
                      n174 = Type Cast(type=dbl[] [] ("array"), x=w491) -> (*(type *) &x=w489:dbl[])
                      n175 = Index Array(array=w489) -> (element #1=w488:dbl, element #2=w487:dbl)  [unwired: 2 in]
                    }
                  }
                }
                frame True {
                  w492 = 0.0
                }
              }
              n176 = call "PH_PPMA_PowerUnit.get data to modify.vi"("i ref in"=w454, "error in (no error)"=w452) -> ("i ref out"=w462:refnum<vi>, "i attribute"=w458:T10, "timed out"=w455:bool, "error out"=w460:errorcluster)  [unwired: 14 in]
              n177 = case shown="False" w455 {
                tunnel: w462 -> [w472 w474]
                tunnel: [w471 w474] -> w461
                tunnel: w460 -> [w470 w473]
                tunnel: [w469 w473] -> w459
                tunnel: w458 -> [w468 _]
                tunnel: w457 -> [w467 _]
                tunnel: w456 -> [w466 _]
                frame False {
                  n178 = Bundle By Name(cluster=w468, "PSU.lower limit [V]"=w467, "PSU.upper limit [V]"=w466) -> (w465:T10)
                  n179 = call "PH_PPMA_PowerUnit.set modified data.vi"("i ref in"=w472, "i attribute"=w465, "error in (no error)"=w470) -> ("i ref out"=w471:refnum<vi>, "error out"=w469:errorcluster)  [unwired: 15 in]
                }
                frame True {
                }
              }
            }
            frame Error {
            }
          }
          n180 = call "BaseProcess.set event status.vi"("i ref in"=w436, "EventStatus"=w444, "error in (no error)"=w435) -> ("i ref out"=w446:refnum<vi>, "error out"=w445:errorcluster)  [unwired: 14 in, 1 out]
          n181 = case shown="No Error" w445 {
            selector: w445 -> [_ w497]
            tunnel: [_ w495] -> w448
            frame No Error {
            }
            frame Error {
              n182 = Unbundle By Name(w497) -> ("source"=w496:string)
              n183 = call-poly "CoreLib.data 2 byte array.vi"("string"=w496) -> ("byteArray out"=w495:T1)  [unwired: 18 in]
            }
          }
          n184 = Unbundle By Name(w445) -> ("code"=w447:i32)
          n185 = Bundle By Name(cluster=w443, "Data"=w448, "Error #"=w447) -> (w442:T2)
        }
        frame "_set_PSDB_Data" {
          n186 = call "CAEObj.unfold trend data.vi"("i ref in"=w501, "raw trend data"=w502) -> ("quality"=w503:i32, "no link"=w506:bool, "data"=w504:i8[], "typeDescriptor"=w505:string, "error out"=w507:errorcluster)  [unwired: 9 in, 4 out]
          n187 = case shown="No Error" w507 {
            tunnel: w500 -> [w524 w560]
            tunnel: [w526 w559] -> w498
            tunnel: [w525 w560] -> w499
            tunnel: w501 -> [w523 w559]
            tunnel: w506 -> [w516 _]
            tunnel: w505 -> [w518 _]
            tunnel: w504 -> [w519 _]
            tunnel: w503 -> [w517 _]
            frame No Error {
              n188 = call "PH_PSDBWriter.get Subsystem DIM Service.vi"("no link"=w516, "typeDescriptor"=w518, "data"=w519, "quality"=w517) -> ("PHELIX Subsystems"=w515:T15)
              n189 = call "PH_PSDBWriter.check PSDB writing condition.vi"("i ref in"=w523, "wanted Subsystem"=w515, "error IO"=w524) -> ("i ref out"=w522:refnum<vi>, "write PSDB?"=w520:bool, "error out"=w521:errorcluster)  [unwired: 14 in]
              n190 = case shown="True" w520 {
                tunnel: w521 -> [w527 w531]
                tunnel: [w528 w534] -> w526
                tunnel: [w527 w535] -> w525
                tunnel: w522 -> [w528 w533]
                frame False {
                }
                frame True {
                  n191 = call "BaseSM.check state.vi"("i ref in"=w533, "error in (no error)"=w531) -> ("i ref out"=w532:refnum<vi>, "actualState"=w529:string, "error out"=w530:errorcluster)  [unwired: 12 in, 3 out]
                  n192 = case shown="\"Stand by\", \"Switch PU on\", \"Wait for Shot Cmd\"" w529 {
                    tunnel: [w541 w557] -> w535
                    tunnel: [w538 w555] -> w534
                    tunnel: w532 -> [w540 w554]
                    tunnel: w530 -> [w543 w553]
                    frame Default {
                      n193 = call "PH_PowerUnit_BaseClass.get data to modify.vi"("i ref in"=w540, "error in (no error)"=w543) -> ("i ref out"=w539:refnum<vi>, "i attribute"=w536:T5, "timed out"=w537:bool, "error out"=w542:errorcluster)  [unwired: 14 in]
                      n194 = case shown="False" w537 {
                        tunnel: w542 -> [w550 w551]
                        tunnel: [w549 w551] -> w541
                        tunnel: w539 -> [w548 w552]
                        tunnel: [w547 w552] -> w538
                        tunnel: w536 -> [w546 _]
                        frame False {
                          n195 = Bundle By Name(cluster=w546, "PSDB data.Write 2 early"=TRUE) -> (w545:T5)
                          n196 = call "PH_PowerUnit_BaseClass.set modified data.vi"("i ref in"=w548, "i attribute"=w545, "error in (no error)"=w550) -> ("i ref out"=w547:refnum<vi>, "error out"=w549:errorcluster)  [unwired: 15 in]
                        }
                        frame True {
                        }
                      }
                    }
                    frame "Stand by", "Switch PU on", "Wait for Shot Cmd" {
                      n197 = call "PH_PPMA_PowerUnit.write PSDB.vi"("i ref in"=w554, "error IO"=w553) -> ("i ref out"=w556:refnum<vi>, "error out"=w558:errorcluster)  [unwired: 16 in]
                      n198 = call "PH_PSDBWriter.evt call write PSDB.vi"("i ref in"=w556, "error in (no error)"=w558) -> ("i ref out"=w555:refnum<vi>, "error out"=w557:errorcluster)  [unwired: 16 in]
                    }
                  }
                }
              }
            }
            frame Error {
            }
          }
          n199 = call "BaseProcess.set event status.vi"("i ref in"=w498, "EventStatus"=w510, "error in (no error)"=w499) -> ("i ref out"=w512:refnum<vi>, "error out"=w511:errorcluster)  [unwired: 14 in, 1 out]
          n200 = Unbundle By Name(w511) -> ("code"=w513:i32)
          n201 = case shown="Error" w511 {
            selector: w511 -> [_ w563]
            tunnel: [_ w561] -> w514
            frame No Error {
            }
            frame Error {
              n202 = Unbundle By Name(w563) -> ("source"=w562:string)
              n203 = call-poly "CoreLib.data 2 byte array.vi"("string"=w562) -> ("byteArray out"=w561:T1)  [unwired: 18 in]
            }
          }
          n204 = Bundle By Name(cluster=w509, "Data"=w514, "Error #"=w513) -> (w508:T2)
        }
        frame "_SMStateSequencer" {
          n205 = call "CAEObj.unfold trend data.vi"("i ref in"=w567, "raw trend data"=w568) -> ("quality"=w569:i32, "no link"=w572:bool, "data"=w570:i8[], "typeDescriptor"=w571:string, "error out"=w573:errorcluster)  [unwired: 9 in, 4 out]
          n206 = case shown="No Error" w573 {
            tunnel: w566 -> [w591 w593]
            tunnel: [w581 w592] -> w564
            tunnel: [w583 w593] -> w565
            tunnel: w567 -> [w590 w592]
            tunnel: w572 -> [w584 _]
            tunnel: w571 -> [w588 _]
            tunnel: w570 -> [w587 _]
            tunnel: w569 -> [w586 _]
            frame No Error {
              n207 = call "PH_DIM.get String.vi"("no link"=w584, "typeDescriptor"=w588, "data"=w587, "quality"=w586) -> ("Output String"=w585:string)
              n208 = call "PH_PowerUnit_BaseClass.PC Seq SM.vi"("i ref in"=w590, "SM State"=w585, "no link"=w584, "error in"=w591) -> ("i ref out"=w582:refnum<vi>, "error out"=w589:errorcluster)  [unwired: 14 in]
              n209 = call "PH_PPMA_PowerUnit.Action Seq SM.vi"("VI in"=w582, "error in (no error)"=w589) -> ("VI out"=w581:refnum<vi>, "error out"=w583:errorcluster)  [unwired: 16 in]
            }
            frame Error {
            }
          }
          n210 = call "BaseProcess.set event status.vi"("i ref in"=w564, "EventStatus"=w576, "error in (no error)"=w565) -> ("i ref out"=w578:refnum<vi>, "error out"=w577:errorcluster)  [unwired: 14 in, 1 out]
          n211 = Unbundle By Name(w577) -> ("code"=w579:i32)
          n212 = case shown="Error" w577 {
            selector: w577 -> [_ w596]
            tunnel: [_ w594] -> w580
            frame No Error {
            }
            frame Error {
              n213 = Unbundle By Name(w596) -> ("source"=w595:string)
              n214 = call-poly "CoreLib.data 2 byte array.vi"("string"=w595) -> ("byteArray out"=w594:T1)  [unwired: 18 in]
            }
          }
          n215 = Bundle By Name(cluster=w575, "Data"=w580, "Error #"=w579) -> (w574:T2)
        }
        frame Default {
          n216 = call "PH_PowerUnit_BaseClass.ProcCases.vi"("i ref in"=w602, "selector"=w603, "Data"=w601, "call cluster"=w604, "error in (no error)"=w606) -> ("i ref out"=w600:refnum<vi>, "answer cluster"=w605:T2, "error out"=w598:errorcluster)  [unwired: 12 in]
          n217 = call "PH_PPMA_PowerUnit.Calc State PU.vi"("i ref in"=w600, "error in (no error)"=w598) -> ("i ref out"=w599:refnum<vi>, "error out"=w597:errorcluster)  [unwired: 16 in]
        }
      }
    }
    frame Error {
    }
  }
  "answer cluster" <- w7
  "i ref out" <- w4
  "error out" <- w3
